vi "1 axis move_copy.vi"(2 "Deceleration":bool, 4 "RESET":bool, 5 "Stop":bool, 6 "Accelaration":bool, 7 "error in (no error)":errorcluster, 8 "A axis":i32, 9 "Comport":refnum<visa-resource-name>) -> (3 "A out":dbl)   [LabVIEW 2020]
uses:
  <vilib>/Instr/_visa.llb/VISA Configure Serial Port (Instr).vi
  GlobalValue.vi
panel:
  out "element":u8
  out "read buffer":string
  # "COMPORT"
  # "To Move"
  # "Moved"
  # "Microns"
  # "Microns"
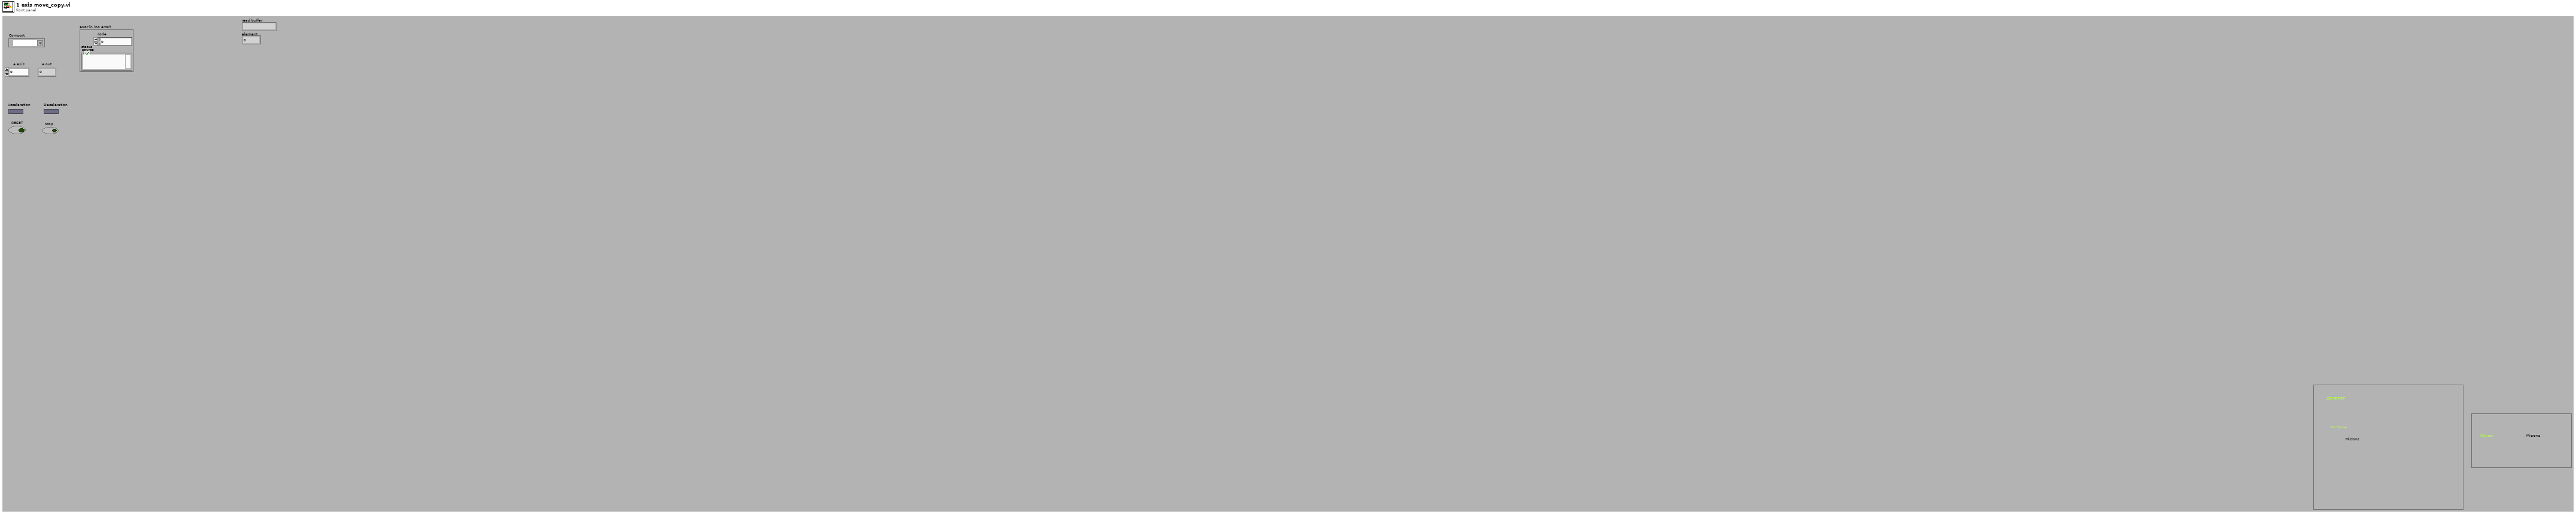
[diagram p1: front panel]
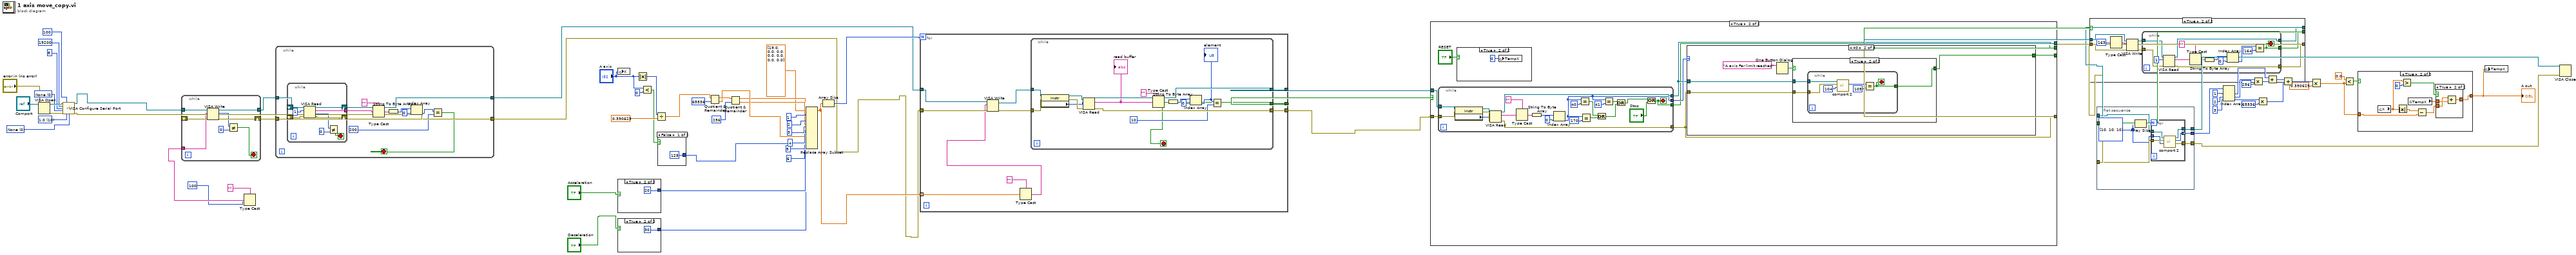
[diagram p0: block diagram]
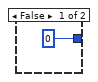
[diagram p2: hidden frame]
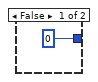
[diagram p3: hidden frame]
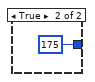
[diagram p4: hidden frame]
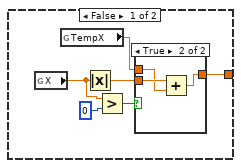
[diagram p5: hidden frame]
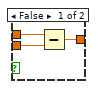
[diagram p6: hidden frame]
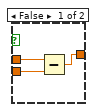
[diagram p7: hidden frame]
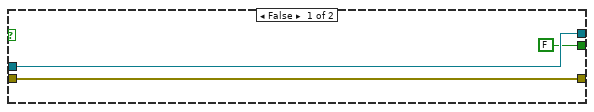
[diagram p8: hidden frame]
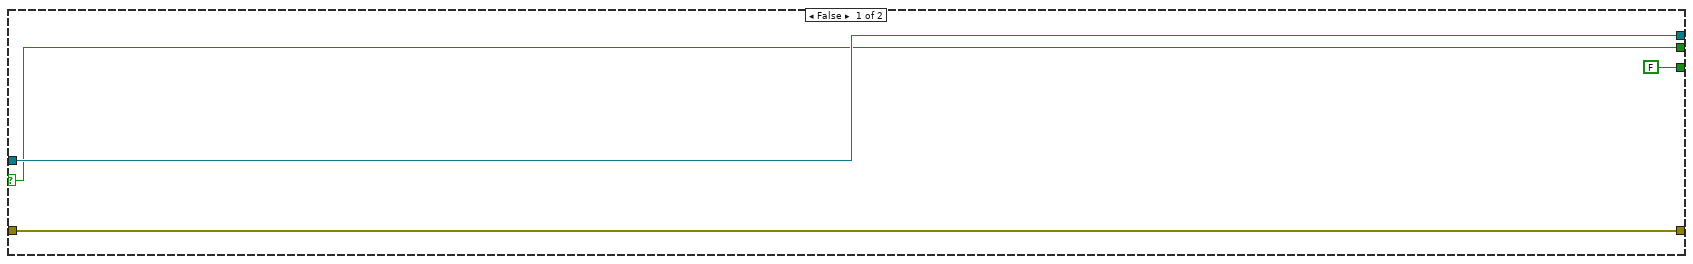
[diagram p9: hidden frame]
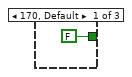
[diagram p11: hidden frame]
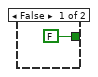
[diagram p12: hidden frame]
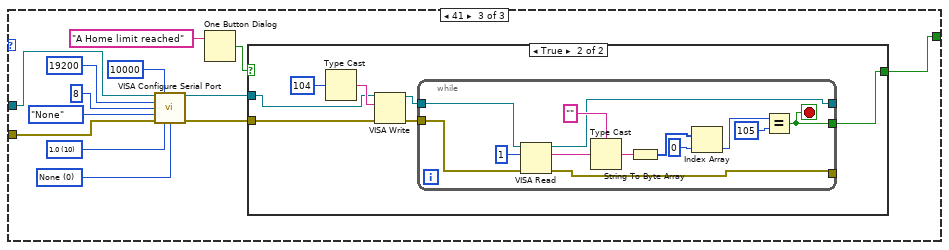
[diagram p13: hidden frame]
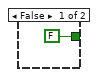
[diagram p14: hidden frame]
diagram:
  w69 = u16 0 items=["None"=0, "XON/XOFF"=1, "RTS/CTS"=2, "DTR/DSR"=4] ("flow control")
  w68 = u16 10 items=["1.0"=10, "1.5"=15, "2.0"=20] ("stop bits")
  w67 = u16 0 items=["None", "Odd", "Even", "Mark", "Space"] ("parity")
  n1 = VISA Open(error in (no error)="error in (no error)", VISA resource name="Comport") -> (VISA resource name=w72:refnum<visa-resource-name>, error out=w73:errorcluster)  [unwired: 3 in]
  n2 = call-poly "VISA Configure Serial Port"("VISA resource name"=w72, "timeout (10sec)"=u32 100, "baud rate (9600)"=u32 19200 ("baud rate"), "data bits (8)"=u16 8 ("data bits"), "parity (0:none)"=w67, "error in (no error)"=w73, "stop bits (10: 1 bit)"=w68, "flow control (0:none)"=w69) -> ("VISA resource name out"=w64:refnum<visa-resource-name>, "error out"=w63:errorcluster)  [unwired: 1 in, 5 out]
  n3 = Type Cast(type="", x=u8 100) -> (*(type *) &x=w28:string)
  n4 = while {
    tunnel: w28 -> [w82]
    shift-right: [w78] -> w25
    shift-left: w63 -> [w80]
    tunnel: w64 -> [w81]
    tunnel: [w79] -> w26
    stop <- w75 stop-if-true
    n5 = VISA Write(VISA resource name=w81, write buffer=w82, error in (no error)=w80) -> (VISA resource name out=w79:refnum<visa-resource-name>, return count=w77:u32, error out=w78:errorcluster)
    n6 = Not Equal?(x=w77, y=u32 0) -> (x != y?=w75:bool)
  }
  n7 = while {
    tunnel: w25 -> [w93]
    tunnel: [w91] -> w31
    tunnel: w26 -> [w94]
    tunnel: [w92] -> w61
    stop <- w86 stop-if-true
    n8 = while {
      tunnel: [w98] -> w85
      shift-right: [w101] -> w92
      shift-left: w94 -> [w103]
      shift-right: [w100] -> w91
      shift-left: w93 -> [w102]
      stop <- w95 stop-if-true
      n9 = VISA Read(VISA resource name=w103, byte count=u32 1, error in (no error)=w102) -> (VISA resource name out=w101:refnum<visa-resource-name>, read buffer=w98:string, return count=w96:u32, error out=w100:errorcluster)
      n10 = Not Equal?(x=w96, y=u32 0) -> (x != y?=w95:bool)
    }
    n11 = Type Cast(type="", x=w85) -> (*(type *) &x=w83:string)
    n12 = String To Byte Array(string=w83) -> (unsigned byte array=w90:u8[])
    n13 = Index Array(array=w90, index=0) -> (element=w88:u8)
    n14 = Equal?(x=w88, y=u8 200) -> (x = y?=w86:bool)
  }
  n15 = global write "GlobalValue.vi" "X"("A axis") -> ()
  n16 = case shown="True" "Accelaration" {
    tunnel: [0 20] -> w15
    frame False {
    }
    frame True {
    }
  }
  n17 = case shown="True" "Deceleration" {
    tunnel: [0 30] -> w13
    frame False {
    }
    frame True {
    }
  }
  n18 = Absolute Value(x="A axis") -> (abs(x)=w20:i32)
  n19 = Less?(x="A axis", y=0) -> (x < y?=w22:bool)
  n20 = Divide(x=w20, y=0.390625) -> (x/y=w8:dbl)
  n21 = case shown="False" w22 {
    tunnel: [u16 125 u16 175] -> w17
    frame False {
    }
    frame True {
    }
  }
  n22 = Quotient & Remainder(x=w8, y=65536) -> (x-y*floor(x/y)=w6:dbl, floor(x/y)=w4:dbl)
  n23 = Quotient & Remainder(x=w6, y=256) -> (x-y*floor(x/y)=w2:dbl, floor(x/y)=w3:dbl)
  n24 = Replace Array Subset(array=dbl[] [19.0, 0.0, 0.0, 0.0, 0.0, 0.0, 0.0], new element #1=w2, index #1=1 ("index"), new element #2=w3, index #2=2 ("index"), new element #3=w4, index #3=3 ("index"), new element #4=w17, index #4=4 ("index"), new element #5=w15, index #5=5 ("index"), new element #6=w13, index #6=6 ("index")) -> (w60:dbl[])
  n25 = Array Size(array=w60) -> (size(s)=w62:i32)
  n26 = for {
    N: w62 -> [_]
    tunnel: [w114] -> w58
    tunnel: w61 -> [w118]
    tunnel: [w116] -> w59
    tunnel: w31 -> [w117]
    tunnel: [w115] -> w30
    tunnel: w60 -> [w111] mode=indexing
    n27 = Type Cast(type="", x=w111) -> (*(type *) &x=w110:string)
    n28 = VISA Write(VISA resource name=w118, write buffer=w110, error in (no error)=w117) -> (VISA resource name out=w113:refnum<visa-resource-name>, error out=w112:errorcluster)  [unwired: 1 out]
    n29 = while {
      tunnel: w112 -> [w123]
      tunnel: [w133] -> w115
      tunnel: w113 -> [w124]
      tunnel: [w134] -> w116
      tunnel: [w128] -> w114
      stop <- w128 stop-if-true
      n30 = property class="Instr"(reference=w124, error in=w123) -> (reference out=w122:refnum<visa-resource-name>, error out=w121:errorcluster, "Serial Settings:Number of Bytes at Serial Port"=w120:u32)
      n31 = VISA Read(VISA resource name=w122, byte count=w120, error in (no error)=w121) -> (VISA resource name out=w134:refnum<visa-resource-name>, read buffer=w127:string, error out=w133:errorcluster)  [unwired: 1 out]
      "read buffer" <- w127
      n32 = Type Cast(type="", x=w127) -> (*(type *) &x=w125:string)
      n33 = String To Byte Array(string=w125) -> (unsigned byte array=w132:u8[])
      n34 = Index Array(array=w132, index=0) -> (element=w130:u8)
      "element" <- w130
      n35 = Equal?(x=w130, y=u8 10) -> (x = y?=w128:bool)
    }
  }
  n36 = case shown="True" w58 {
    selector: w58 -> [w135 _]
    tunnel: w59 -> [w138 w143]
    tunnel: w30 -> [w137 w145]
    tunnel: [w138 w142] -> w57
    tunnel: [w137 w141] -> w55
    tunnel: [w135 w139] -> w56
    tunnel: [FALSE w140] -> _
    frame False {
    }
    frame True {
      n37 = while {
        tunnel: w145 -> [w150]
        tunnel: [w156] -> w142
        tunnel: [w159] -> w141
        tunnel: [w158] -> w139
        tunnel: [w155] -> w144
        tunnel: w143 -> [w151]
        stop <- w158 stop-if-true
        n38 = property class="Instr"(reference=w151, error in=w150) -> (reference out=w149:refnum<visa-resource-name>, error out=w148:errorcluster, "Serial Settings:Number of Bytes at Serial Port"=w147:u32)
        n39 = VISA Read(VISA resource name=w149, byte count=w147, error in (no error)=w148) -> (VISA resource name out=w156:refnum<visa-resource-name>, read buffer=w168:string, error out=w159:errorcluster)  [unwired: 1 out]
        n40 = Type Cast(type="", x=w168) -> (*(type *) &x=w169:string)
        n41 = String To Byte Array(string=w169) -> (unsigned byte array=w167:u8[])
        n42 = Index Array(array=w167, index=0) -> (element=w155:u8)
        n43 = Equal?(x=w155, y=u8 40) -> (x = y?=w154:bool)
        n44 = Equal?(x=w155, y=u8 170) -> (x = y?=w157:bool)
        n45 = Or(x=w154, y=w157) -> (x .or. y?=w153:bool)
        n46 = Equal?(x=w155, y=u8 41) -> (x = y?=w162:bool)
        n47 = Or(x=w162, y=w153) -> (x .or. y?=w152:bool)
        n48 = Or(x=w152, y="Stop") -> (x .or. y?=w158:bool)
      }
      n49 = case shown="True" "RESET" {
        frame False {
        }
        frame True {
          n50 = global write "GlobalValue.vi" "TempX"(0) -> ()
        }
      }
      n51 = case shown="40" w144 {
        tunnel: w142 -> [_ w173 w196]
        tunnel: w141 -> [_ w174 w193]
        tunnel: [FALSE w172 w197] -> w140
        frame 170, Default {
        }
        frame 40 {
          n52 = One Button Dialog(message="A axis Far limit reached") -> (true=w175:bool)  [unwired: 1 in]
          n53 = case shown="True" w175 {
            tunnel: w174 -> [_ w179]
            tunnel: w173 -> [_ w180]
            tunnel: [FALSE w178] -> w172
            frame False {
            }
            frame True {
              n54 = while {
                tunnel: w180 -> [w186]
                tunnel: w179 -> [w185]
                tunnel: [w181] -> w178
                stop <- w181 stop-if-true
                n55 = call "comport 2.vi"("x"=u8 104, "error in (no error)"=w185, "VISA resource name"=w186) -> ("Numeric"=w183:u8)  [unwired: 6 in, 2 out]
                n56 = Equal?(x=w183, y=u8 105) -> (x = y?=w181:bool)
              }
            }
          }
        }
        frame 41 {
          w188 = u16 0 items=["None", "XON/XOFF", "RTS/CTS", "XON/XOFF & RTS/CTS", "DTR/DSR", "XON/XOFF & DTR/DSR"] ("flow control (0:none)")
          w189 = u16 10 items=["1.0"=10, "1.5"=15, "2.0"=20] ("stop bits (10: 1 bit)")
          n57 = call-poly "VISA Configure Serial Port"("VISA resource name"=w196, "timeout (10sec)"=u32 10000, "baud rate (9600)"=u32 19200, "data bits (8)"=u16 8, "parity (0:none)"=enum16{"None", "Odd", "Even", "Mark", "Space"}."None", "error in (no error)"=w193, "stop bits (10: 1 bit)"=w189, "flow control (0:none)"=w188) -> ("VISA resource name out"=w195:refnum<visa-resource-name>, "error out"=w194:errorcluster)  [unwired: 6 in]
          n58 = One Button Dialog(message="A Home limit reached") -> (true=w198:bool)  [unwired: 1 in]
          n59 = case shown="True" w198 {
            tunnel: w195 -> [_ w204]
            tunnel: w194 -> [_ w203]
            tunnel: [FALSE w201] -> w197
            frame False {
            }
            frame True {
              n60 = Type Cast(x=104) -> (*(type *) &x=w207:string)  [unwired: 1 in]
              n61 = VISA Write(VISA resource name=w204, write buffer=w207, error in (no error)=w203) -> (VISA resource name out=w205:refnum<visa-resource-name>, error out=w206:errorcluster)  [unwired: 1 out]
              n62 = while {
                tunnel: w206 -> [w220]
                tunnel: [w210] -> _
                tunnel: w205 -> [w219]
                tunnel: [w209] -> _
                tunnel: [w208] -> w201
                stop <- w208 stop-if-true
                n63 = VISA Read(VISA resource name=w219, byte count=u32 1, error in (no error)=w220) -> (VISA resource name out=w209:refnum<visa-resource-name>, read buffer=w211:string, error out=w210:errorcluster)  [unwired: 1 out]
                n64 = Type Cast(type="", x=w211) -> (*(type *) &x=w212:string)
                n65 = String To Byte Array(string=w212) -> (unsigned byte array=w216:u8[])
                n66 = Index Array(array=w216, index=0) -> (element=w213:u8)
                n67 = Equal?(x=w213, y=u8 105) -> (x = y?=w208:bool)
              }
            }
          }
        }
      }
    }
  }
  n68 = case shown="True" w56 {
    tunnel: w57 -> [w223 w229]
    tunnel: w55 -> [w222 w228]
    tunnel: [FALSE w227] -> w32
    tunnel: [w223 w225] -> w54
    tunnel: [w222 w226] -> w53
    frame False {
    }
    frame True {
      n69 = Type Cast(x=163) -> (*(type *) &x=w232:string)  [unwired: 1 in]
      n70 = VISA Write(VISA resource name=w229, write buffer=w232, error in (no error)=w228) -> (VISA resource name out=w230:refnum<visa-resource-name>, error out=w231:errorcluster)  [unwired: 1 out]
      n71 = while {
        tunnel: w231 -> [w245]
        tunnel: [w235] -> w226
        tunnel: w230 -> [w244]
        tunnel: [w234] -> w227
        tunnel: [w233] -> w225
        stop <- w234 stop-if-true
        n72 = VISA Read(VISA resource name=w244, byte count=u32 1, error in (no error)=w245) -> (VISA resource name out=w233:refnum<visa-resource-name>, read buffer=w236:string, error out=w235:errorcluster)  [unwired: 1 out]
        n73 = Type Cast(type="", x=w236) -> (*(type *) &x=w237:string)
        n74 = String To Byte Array(string=w237) -> (unsigned byte array=w241:u8[])
        n75 = Index Array(array=w241, index=0) -> (element=w238:u8)
        n76 = Equal?(x=w238, y=u8 164) -> (x = y?=w234:bool)
      }
    }
  }
  n77 = flat-sequence {
    tunnel: w53 -> [w251]
    tunnel: [w249] -> w51
    tunnel: [w250] -> w52
    tunnel: w54 -> [w248]
    tunnel: [w247] -> w50
    tunnel: w32 -> [_]
    frame #0 {
      w246 = u8[] [10, 10, 10]
      n78 = Array Size(array=w246) -> (size(s)=w252:i32)
      n79 = for {
        N: w252 -> [_]
        tunnel: w251 -> [w256]
        tunnel: [w257] -> w250
        tunnel: w248 -> [w258]
        tunnel: [w253] -> w249
        tunnel: [w254] -> w247 mode=indexing
        tunnel: w246 -> [w255] mode=indexing
        n80 = call "comport 2.vi"("x"=w255, "error in (no error)"=w256, "VISA resource name"=w258) -> ("error out"=w253:errorcluster, "Numeric"=w254:u8, "VISA resource name out"=w257:refnum<visa-resource-name>)  [unwired: 6 in]
      }
    }
  }
  n81 = Index Array(array=w50, index #1=1 ("index"), index #2=2 ("index"), index #3=3 ("index")) -> (element #1=w35:u8, element #2=w34:u8, element #3=w33:u8)
  n82 = Multiply(x=w34, y=u16 256) -> (x*y=w45:u16)
  n83 = Multiply(x=w33, y=u32 65536) -> (x*y=w44:u32)
  n84 = Add(x=w35, y=w45) -> (x+y=w43:u16)
  n85 = Add(x=w43, y=w44) -> (x+y=w39:u32)
  n86 = Multiply(x=w39, y=0.390625) -> (x*y=w40:dbl)
  n87 = Less?(x=0.0, y=w40) -> (x < y?=w41:bool)
  n88 = case shown="True" w41 {
    tunnel: w40 -> [_ w278]
    tunnel: [w261 w273] -> w49
    frame False {
      n89 = global read "GlobalValue.vi" "X"() -> (w260:dbl)
      n90 = global read "GlobalValue.vi" "TempX"() -> (w262:dbl)
      n91 = Absolute Value(x=w260) -> (abs(x)=w259:dbl)
      n92 = Greater?(x=w260, y=0) -> (0:w263:bool)
      n93 = case shown="True" w263 {
        tunnel: w259 -> [w266 w270]
        tunnel: w262 -> [w267 w269]
        tunnel: [w265 w268] -> w261
        frame False {
          n94 = Subtract(x=w267, y=w266) -> (x-y=w265:dbl)
        }
        frame True {
          n95 = Add(x=w270, y=w269) -> (x+y=w268:dbl)
        }
      }
    }
    frame True {
      n96 = global read "GlobalValue.vi" "X"() -> (w272:dbl)
      n97 = Absolute Value(x=w272) -> (abs(x)=w271:dbl)
      n98 = Greater?(x=w272, y=0) -> (0:w276:bool)
      n99 = global read "GlobalValue.vi" "TempX"() -> (w274:dbl)
      n100 = Subtract(x=w271, y=w278) -> (x-y=w275:dbl)
      n101 = case shown="True" w276 {
        tunnel: w275 -> [w280 w284]
        tunnel: w274 -> [w281 w283]
        tunnel: [w279 w282] -> w273
        frame False {
          n102 = Subtract(x=w281, y=w280) -> (x-y=w279:dbl)
        }
        frame True {
          n103 = Add(x=w284, y=w283) -> (x+y=w282:dbl)
        }
      }
    }
  }
  "A out" <- w49
  n104 = global write "GlobalValue.vi" "TempX"(w49) -> ()
  n105 = VISA Close(VISA resource name=w52, error in (no error)=w51) -> ()  [unwired: 1 out]
